vi "Salvar_Carregar.vi"(7 "LabVIEW Web Service Request":refnum<class "Web Request.lvclass">) -> ()   [LabVIEW 2020]
uses:
  <vilib>/wsapi/Web Request.lvclass
  4e0f3b2c-ee5c-4a40-9e8d-f2c59b176449.vi
panel:
  in  "Operacao":i32
  # "Use the Web Service Request input terminal to call the VIs on the Web Services palette. Do not remove it from the connector pane unless you don't need access to the palette."
  # "Each additional control wired to the connector pane will be available as an input in the URL. To include an indicator in terminal-mode output (the default setting), it must also be wired to the connector pane."
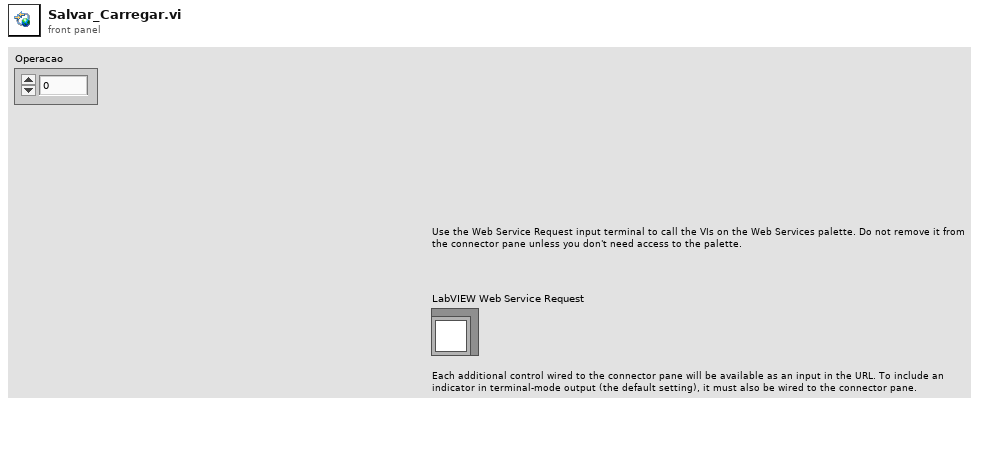
[diagram p1: front panel]
types:
  T1 = enum16{"create", "fire - Simular onda", "fire - Editar onda", "fire - Salvar ou carregar onda", "destroy"}
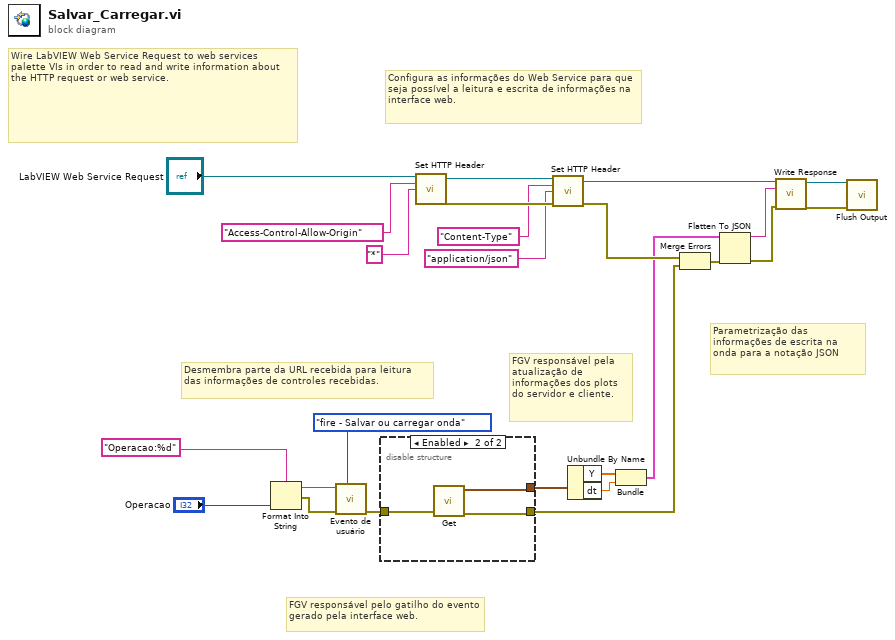
[diagram p0: block diagram]
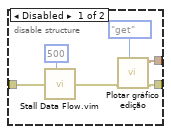
[diagram p2: hidden frame]
diagram:
  # "Parametrização das informações de escrita na onda para a notação JSON"
  # "FGV responsável pela atualização de informações dos plots do servidor e cliente."
  # "FGV responsável pelo gatilho do evento gerado pela interface web."
  # "Desmembra parte da URL recebida para leitura das informações de controles recebidas."
  # "Configura as informações do Web Service para que seja possível a leitura e escrita de informações na interface web."
  # "Wire LabVIEW Web Service Request to web services palette VIs in order to read and write information about the HTTP request or web service."
  n1 = Format Into String(format string="Operacao:%d", "Operacao") -> (resulting string=w15:string, error out=w13:errorcluster)  [unwired: 2 in]
  n2 = call "Evento de usuário.vi"("Enum"=T1."fire - Salvar ou carregar onda", "error in (no error)"=w13, "Dados"=w15) -> ("error out"=w14:errorcluster)  [unwired: 7 in, 1 out]
  n3 = disable-structure shown="Enabled" {
    disable-tunnel: w14 -> [w30 w34]
    disable-tunnel: [w28 w33] -> w7
    disable-tunnel: [w27 w32] -> w6
    frame Disabled {
      n4 = call "Stall Data Flow.vim"("value in"=w30, "milliseconds to wait"=u32 500) -> ("value out"=w29:errorcluster)  [unwired: 1 out]
      n5 = call "Plotar gráfico edição.vi"("Enum"=enum16{"set", "get"}."get", "error in (no error)"=w29) -> ("error out"=w28:errorcluster, "Plot"=w27:waveform(dbl))  [unwired: 8 in]
    }
    frame Enabled {
      n6 = call "Get.vi"("error in"=w34) -> ("error out"=w33:errorcluster, "Waveform In"=w32:waveform(dbl))  [unwired: 9 in]
    }
  }
  n7 = call <vilib>:"Set HTTP Header.vi"("LabVIEW Web Service Request"="LabVIEW Web Service Request", "header"="Access-Control-Allow-Origin", "header value"="*") -> ("LabVIEW Web Service Request out"=w25:refnum<class "Web Request.lvclass">, "error out"=w24:errorcluster)  [unwired: 11 in]
  n8 = call <vilib>:"Set HTTP Header.vi"("LabVIEW Web Service Request"=w25, "header"="Content-Type", "header value"="application/json", "error in (no error)"=w24) -> ("LabVIEW Web Service Request out"=w23:refnum<class "Web Request.lvclass">, "error out"=w12:errorcluster)  [unwired: 10 in]
  n9 = Unbundle By Name(w6) -> ("Y"=w11:dbl[], "dt"=w10:dbl)
  n10 = Bundle("Y"=w11, "dt"=w10) -> (w9:cluster{"Y":dbl[], "dt":dbl})  [unwired: 1 in]
  n11 = Merge Errors(w12, w7) -> (w8:errorcluster)
  n12 = Flatten To JSON(anything=w9, error in (no error)=w8) -> (JSON string=w16:string, 11:w4:errorcluster)  [unwired: 1 in]
  n13 = call <vilib>:"Write Response.vi"("LabVIEW Web Service Request"=w23, "response string"=w16, "error in (no error)"=w4) -> ("LabVIEW Web Service Request out"=w18:refnum<class "Web Request.lvclass">, "error out"=w17:errorcluster)  [unwired: 11 in]
  n14 = call <vilib>:"Flush Output.vi"("LabVIEW Web Service Request"=w18, "error in (no error)"=w17) -> ()  [unwired: 12 in, 2 out]
